vi "14-2.vi"() -> ()   [LabVIEW 2019, in "14.lvlib"]
uses:
  14.lvlib
  <userlib>/_OpenG.lib/array/array.llb/Remove Duplicates from 1D Array (String)__ogtk.vi
panel:
  out "Output Array":string[](array[string])
  out "Array":u64[](array[numeric])
  in  "Steps":i32=2
  out "difference":u64
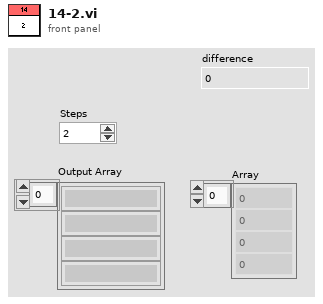
[diagram p1: front panel]
types:
  T1 = cluster{"occurances":u64, "next occurances":u64, "1st replacement":i32, "2nd replacement":i32, "replacement":i32}
  T2 = cluster{"occurances":u64, "next occurances":u64, "1st replacement":i32, "2nd replacement":i32, "replacement":i32}[]
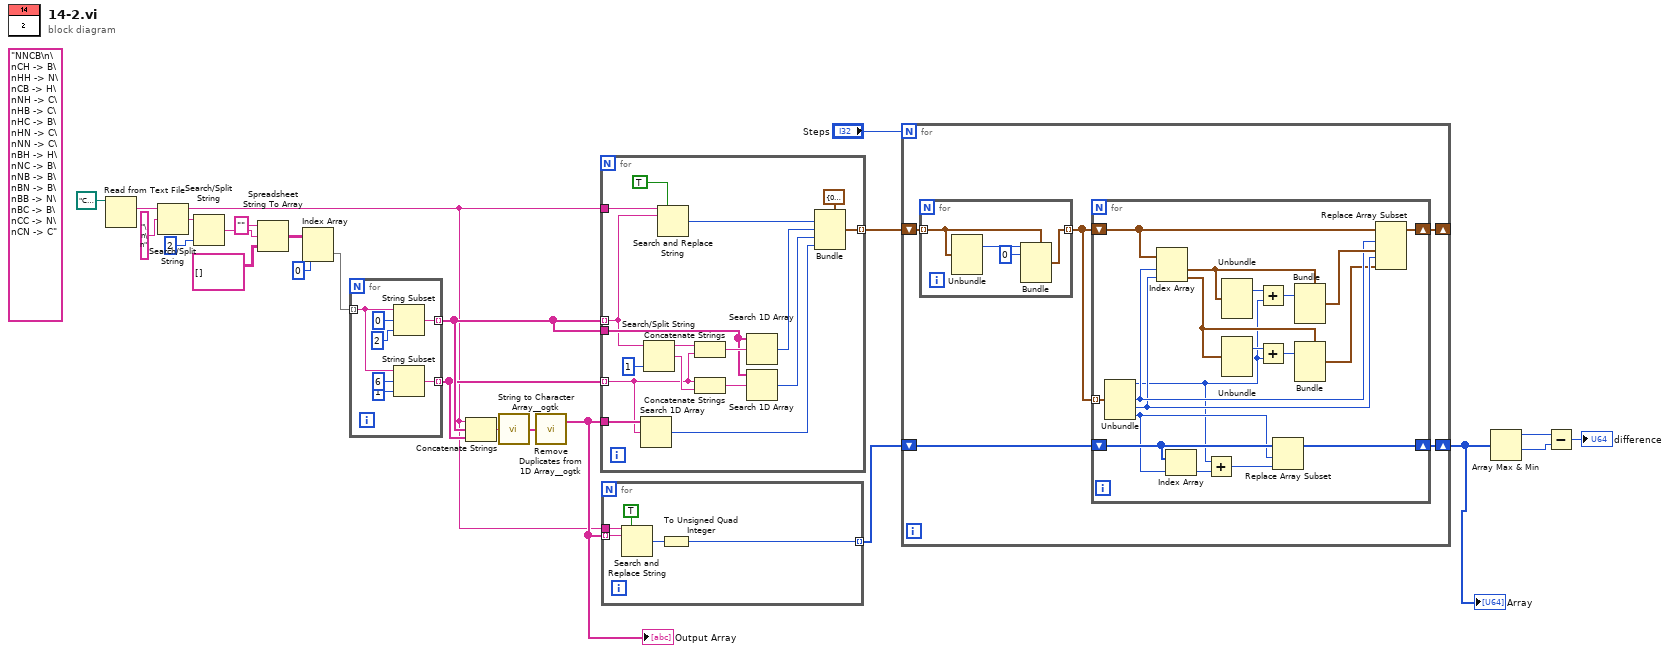
[diagram p0: block diagram]
diagram:
  (unwired) "NNCB\n\nCH -> B\nHH -> N\nCB -> H\nNH -> C\nHB -> C\nHC -> B\nHN -> C\nNN -> C\nBH -> H\nNC -> B\nNB -> B\nBN -> B\nBB -> N\nBC -> B\nCC -> N\nCN -> C"
  n1 = Read from Text File(file (use dialog)=path "C:/Users/craig.walker/Documents/GitHub/lv2019-Advent-of-Code-2021/14/input.txt") -> (text=w1:string)  [unwired: 3 in, 3 out]
  n2 = Search/Split String(string=w1, search string/char (-)="\n\n") -> (substring before match=w7:string, match + rest of string=w22:string)  [unwired: 1 in, 1 out]
  n3 = Search/Split String(string=w22, offset (0)=2) -> (match + rest of string=w20:string)  [unwired: 1 in, 2 out]
  n4 = Spreadsheet String To Array(format string="", spreadsheet string=w20, array type (2D Dbl)=string[][] [] ("search string/char (-)")) -> (array=w18:string[][])  [unwired: 1 in]
  n5 = Index Array(array=w18, index (col)=0 ("disabled index (col)")) -> (element=w15:string[])  [unwired: 1 in]
  n6 = for {
    tunnel: w15 -> [w29] mode=indexing
    tunnel: [w25] -> w12 mode=indexing
    tunnel: [w26] -> w11 mode=indexing
    n7 = String Subset(string=w29, offset (0)=0, length (rest)=2 ("length (rest)")) -> (substring=w25:string)
    n8 = String Subset(string=w29, offset (0)=6, length (rest)=1 ("length (rest)")) -> (substring=w26:string)
  }
  n9 = Concatenate Strings(w7, w12, w11) -> (w10:string)
  n10 = call <userlib>:"String to Character Array__ogtk.vi"("Input String"=w10) -> ("Character Array"=w9:string[])
  n11 = call-poly <userlib>:"Remove Duplicates from 1D Array__ogtk.vi"("Input Array"=w9) -> ("Output Array"=w8:string[])  [unwired: 1 out]
  "Output Array" <- w8
  n12 = for {
    tunnel: w12 -> [w42] mode=indexing
    tunnel: w11 -> [w34] mode=indexing
    tunnel: w12 -> [w44]
    tunnel: w7 -> [w41]
    tunnel: [w38] -> w13 mode=indexing
    tunnel: w8 -> [w35]
    n13 = Search 1D Array(1D array=w35, element=w34) -> (index of element=w33:i32)  [unwired: 1 in]
    n14 = Search/Split String(string=w42, offset (0)=1) -> (substring before match=w47:string, match + rest of string=w46:string)  [unwired: 1 in, 1 out]
    n15 = Search and Replace String(replace all?=TRUE ("replace all? (F)"), input string=w41, search string=w42) -> (number of replacements=w32:i32)  [unwired: 5 in, 3 out]
    n16 = Concatenate Strings(w47, w34) -> (w45:string)
    n17 = Concatenate Strings(w34, w46) -> (w43:string)
    n18 = Search 1D Array(1D array=w44, element=w45) -> (index of element=w36:i32)  [unwired: 1 in]
    n19 = Search 1D Array(1D array=w44, element=w43) -> (index of element=w37:i32)  [unwired: 1 in]
    n20 = Bundle(cluster=T1 {"occurances"=0, "next occurances"=0, "1st replacement"=0, "2nd replacement"=0, "replacement"=0}, "next occurances"=w32, "1st replacement"=w36, "2nd replacement"=w37, "replacement"=w33) -> (w38:T1)  [unwired: 1 in]
  }
  n21 = for {
    tunnel: w8 -> [w52] mode=indexing
    tunnel: w7 -> [w53]
    tunnel: [w49] -> w3 mode=indexing
    n22 = Search and Replace String(replace all?=TRUE ("replace all? (F)"), input string=w53, search string=w52) -> (number of replacements=w50:i32)  [unwired: 5 in, 3 out]
    n23 = To Unsigned Quad Integer(1:w50) -> (0:w49:u64)
  }
  n24 = for {
    N: "Steps" -> [_]
    shift-right: [w56] -> _
    shift-left: w13 -> [w58]
    shift-right: [w55] -> w2
    shift-left: w3 -> [w54]
    n25 = for {
      tunnel: w58 -> [w62] mode=indexing
      tunnel: [w61] -> w57 mode=indexing
      n26 = Unbundle(w62) -> ("next occurances"=w60:u64)  [unwired: 4 out]
      n27 = Bundle(cluster=w62, "occurances"=w60, "next occurances"=u64 0) -> (w61:T1)  [unwired: 3 in]
    }
    n28 = for {
      tunnel: w57 -> [w79] mode=indexing
      shift-right: [w81] -> w56
      shift-left: w57 -> [w78]
      shift-right: [w67] -> w55
      shift-left: w54 -> [w68]
      n29 = Unbundle(w79) -> ("occurances"=w64:u64, "1st replacement"=w75:i32, "2nd replacement"=w74:i32, "replacement"=w66:i32)  [unwired: 1 out]
      n30 = Index Array(array=w78, index #1=w75, index #2=w74) -> (element #1=w77:T1, element #2=w69:T1)
      n31 = Index Array(array=w68, index=w66) -> (element=w65:u64)
      n32 = Add(x=w64, y=w65) -> (x+y=w63:u64)
      n33 = Unbundle(w77) -> ("next occurances"=w76:u64)  [unwired: 4 out]
      n34 = Unbundle(w69) -> ("next occurances"=w71:u64)  [unwired: 4 out]
      n35 = Add(x=w76, y=w64) -> (x+y=w73:u64)
      n36 = Add(x=w71, y=w64) -> (x+y=w72:u64)
      n37 = Replace Array Subset(array=w68, new element=w63, index=w66) -> (w67:u64[])
      n38 = Bundle(cluster=w77, "next occurances"=w73) -> (w80:T1)  [unwired: 4 in]
      n39 = Bundle(cluster=w69, "next occurances"=w72) -> (w70:T1)  [unwired: 4 in]
      n40 = Replace Array Subset(array=w78, new element #1=w80, index #1=w75, new element #2=w70, index #2=w74) -> (w81:T2)
    }
  }
  "Array" <- w2
  n41 = Array Max & Min(array=w2) -> (max value=w6:u64, min value=w5:u64)  [unwired: 2 out]
  n42 = Subtract(x=w6, y=w5) -> (x-y=→"difference":u64)
